vi "About Coleman Technologies.vi"() -> ()   [LabVIEW 2013]
doc: "Gives contact information about Coleman Technologies, Inc."
uses:
  <vilib>/Utility/miscctls.llb/LVPointTypeDef.ctl
  <vilib>/Platform/browser.llb/Open URL in Default Browser (string).vi
panel:
  in  "hyperlink":bool
  in  "End 2":bool
  in  "End":bool
  # "5131 West Chester Pike\nWest Chester, PA 19382\n\nVoice: (610) 459-9646"
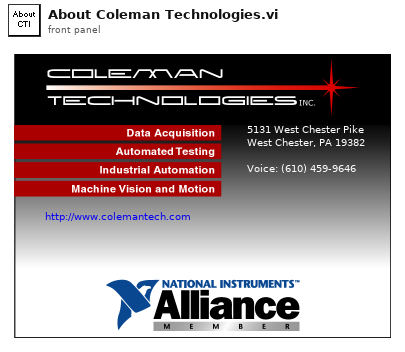
[diagram p1: front panel]
types:
  T1 = typedef "LVPointTypeDef.ctl" = cluster{"Horizontal":i16, "Vertical":i16}
  T2 = enum32{"Bad", "Idle", "Run top level", "Running"}
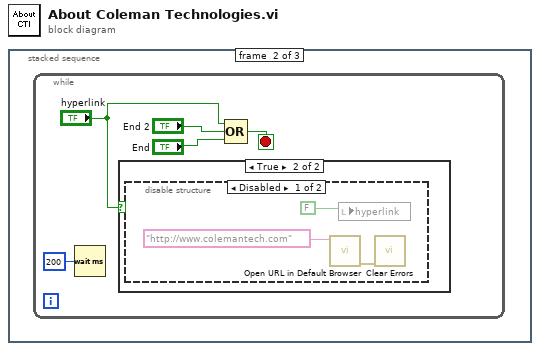
[diagram p0: block diagram]
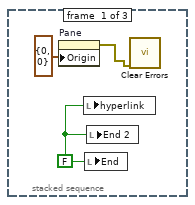
[diagram p2: hidden frame]
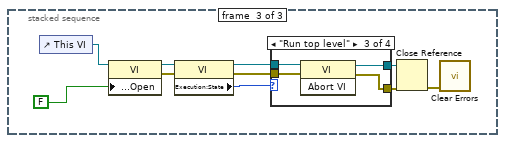
[diagram p5: hidden frame]
diagram:
  n1 = stacked-sequence {
    frame #0 {
      w2 = FALSE ("End")
      n2 = property on="Pane" class="Pane"("Origin"=T1 {"Horizontal"=0, "Vertical"=0}) -> (error out=w1:errorcluster)  [unwired: 2 in, 1 out]
      n3 = local write "hyperlink"(w2) -> ()
      n4 = local write "End"(w2) -> ()
      n5 = local write "End 2"(w2) -> ()
      n6 = call <vilib>:"Clear Errors.vi"("error in (no error)"=w1) -> ()  [unwired: 7 out]
    }
    frame #1 {
      n7 = while {
        stop <- w5 stop-if-true
        n8 = Wait (ms)(milliseconds to wait=u32 200) -> ()  [unwired: 1 out]
        n9 = case shown="True" "hyperlink" {
          frame False {
          }
          frame True {
            n10 = disable-structure shown="Disabled" {
              frame Disabled {
                n11 = call-poly <vilib>:"Open URL in Default Browser.vi"("URL"="http://www.colemantech.com") -> ("error out"=w10:errorcluster)  [unwired: 1 in, 5 out]
                n12 = local write "hyperlink"(FALSE ("Hyperlink")) -> ()
                n13 = call <vilib>:"Clear Errors.vi"("error in (no error)"=w10) -> ()  [unwired: 7 out]
              }
              frame Enabled {
              }
            }
          }
        }
        n14 = Compound Arithmetic op=OR("hyperlink", "End 2", "End") -> (w5:bool)
      }
    }
    frame #2 {
      n15 = control-ref of="This VI"() -> (w13:refnum<vi>)
      n16 = property class="VI"(reference=w13, "Front Panel Window:Open"=FALSE ("FPWindOpen")) -> (reference out=w18:refnum<vi>, error out=w17:errorcluster)  [unwired: 1 in]
      n17 = property class="VI"(reference=w18, error in=w17) -> (reference out=w15:refnum<vi>, error out=w20:errorcluster, "Execution:State"=w21:T2)
      n18 = case shown="\"Run top level\"" w21 {
        tunnel: w20 -> [w23 w25 w28 w31]
        tunnel: [w23 w25 w26 w31] -> w16
        tunnel: w15 -> [w22 w24 w29 w30]
        tunnel: [w22 w24 w27 w30] -> w14
        frame "Bad", Default {
        }
        frame "Idle" {
        }
        frame "Run top level" {
          n19 = invoke class="VI" method="Abort VI"(reference=w29, error in=w28) -> (reference out=w27:refnum<vi>, error out=w26:errorcluster)  [unwired: 1 in, 1 out]
        }
        frame "Running" {
        }
      }
      n20 = Close Reference(reference=w14, error in (no error)=w16) -> (error out=w12:errorcluster)
      n21 = call <vilib>:"Clear Errors.vi"("error in (no error)"=w12) -> ()  [unwired: 7 out]
    }
  }
